vi "Vacuum Test - Step 3.vi"(7 "Step":i32, 8 "error in":errorcluster, 9 "Test Results In":T9, 10 "PAS In":T8 caption="Gas", 11 "Test Configuration":T1) -> (0 "error out":errorcluster, 1 "Test Results Out":T9, 2 "PAS Out":T8 caption="Gas", 3 "Test Configuration Out":T1)   [LabVIEW 2015]
uses:
  CAN Communication/PAS/Typedefs/Session Handle.ctl
  CAN Communication/PAS/PAS.lvclass
  Controls/Test Results.ctl
  Controls/Step Result.ctl
  Controls/Test Configuration.ctl
  Controls/Vacuum Test.ctl
  Controls/Test Timing.ctl
  Controls/Vaccum Thresholds.ctl
  Controls/Helium Test.ctl
  Controls/Helium Thresholds.ctl
  Controls/Functional Test.ctl
  CAN Communication/PAS/Typedefs/Valves.ctl
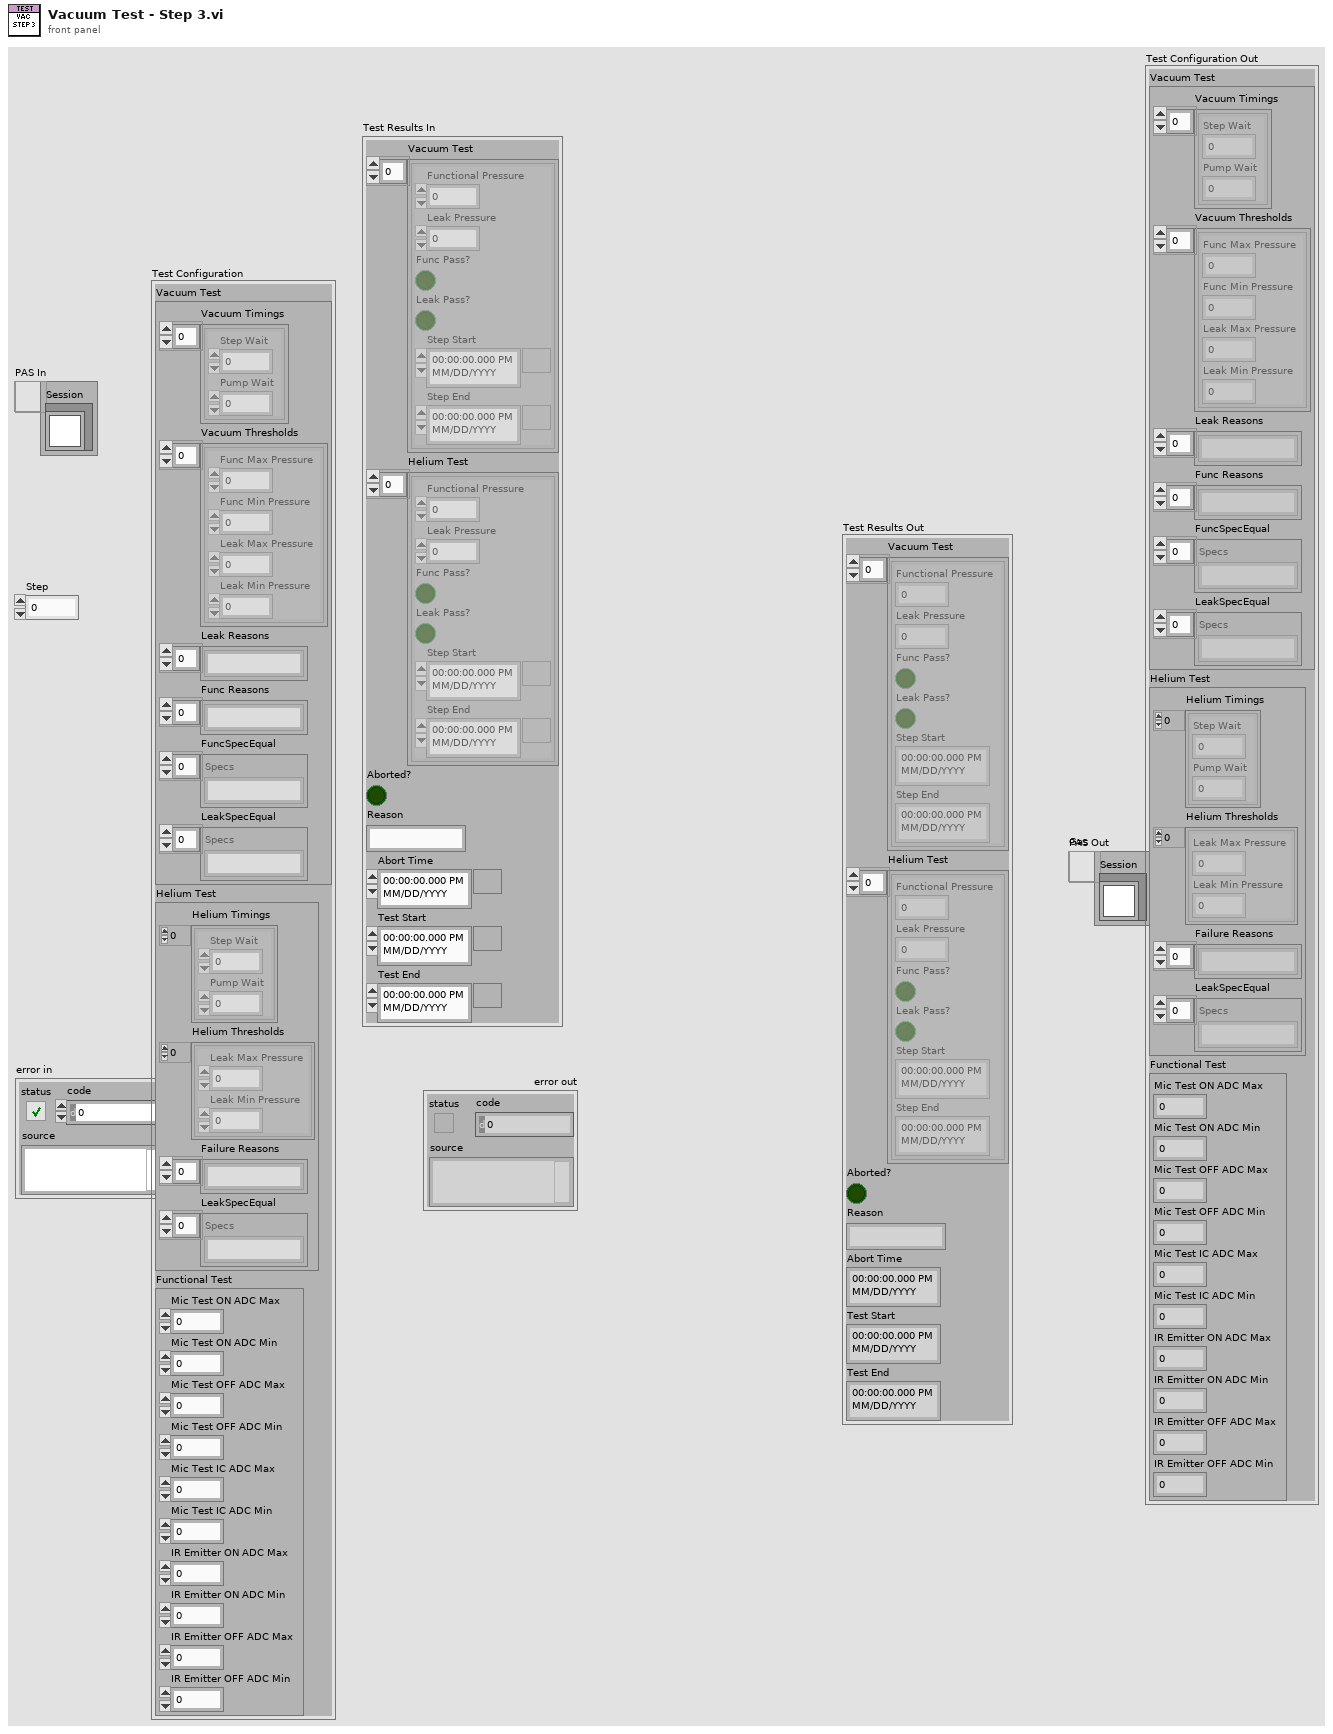
[diagram p1: front panel]
types:
  T1 = typedef "Test Configuration.ctl" = cluster{"Vacuum Test":T2, "Helium Test":T5, "Functional Test":T7}
  T2 = typedef "Vacuum Test.ctl" = cluster{"Vacuum Timings":T3[], "Vacuum Thresholds":T4[], "Leak Reasons":string[], "Func Reasons":string[], "FuncSpecEqual":string[], "LeakSpecEqual":string[]}
  T3 = typedef "Test Timing.ctl" = cluster{"Step Wait":dbl, "Pump Wait":dbl}
  T4 = typedef "Vaccum Thresholds.ctl" = cluster{"Func Max Pressure":dbl, "Func Min Pressure":dbl, "Leak Max Pressure":dbl, "Leak Min Pressure":dbl}
  T5 = typedef "Helium Test.ctl" = cluster{"Helium Timings":T3[], "Helium Thresholds":T6[], "Failure Reasons":string[], "LeakSpecEqual":string[]}
  T6 = typedef "Helium Thresholds.ctl" = cluster{"Leak Max Pressure":dbl, "Leak Min Pressure":dbl}
  T7 = typedef "Functional Test.ctl" = cluster{"Mic Test ON ADC Max":dbl, "Mic Test ON ADC Min":dbl, "Mic Test OFF ADC Max":dbl, "Mic Test OFF ADC Min":dbl, "Mic Test IC ADC Max":dbl, "Mic Test IC ADC Min":dbl, "IR Emitter ON ADC Max":dbl, "IR Emitter ON ADC Min":dbl, "IR Emitter OFF ADC Max":dbl, "IR Emitter OFF ADC Min":dbl}
  T8 = typedef "PAS.lvclass/Session Handle.ctl" = refnum<data-value>
  T9 = typedef "Test Results.ctl" = cluster{"Vacuum Test":T10[], "Helium Test":T10[], "Aborted?":bool, "Reason":string, "Abort Time":timestamp, "Test Start":timestamp, "Test End":timestamp}
  T10 = typedef "Step Result.ctl" = cluster{"Functional Pressure":dbl, "Leak Pressure":dbl, "Func Pass?":bool, "Leak Pass?":bool, "Step Start":timestamp, "Step End":timestamp}
  T11 = typedef "PAS.lvclass/Valves.ctl" = u16
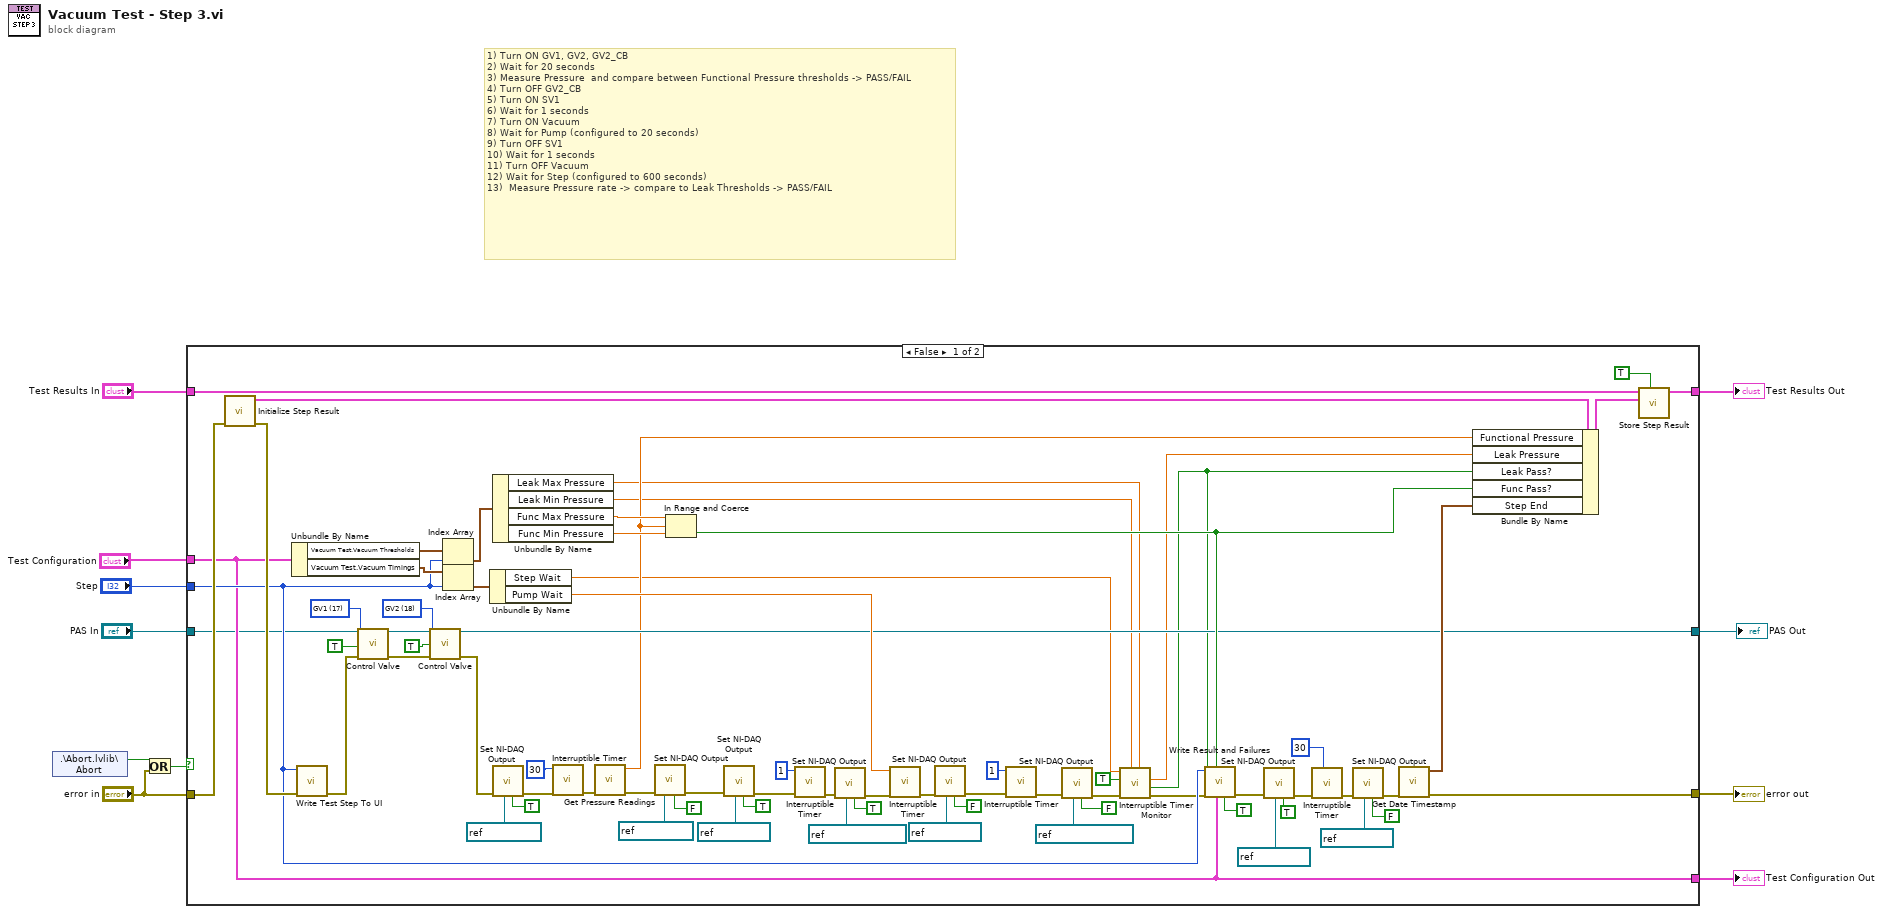
[diagram p0: block diagram]
diagram:
  # "1) Turn ON GV1, GV2, GV2_CB\n2) Wait for 20 seconds\n3) Measure Pressure  and compare between Functional Pressure thresholds -> PASS/FAIL\n4) Turn OFF GV2_CB\n5) Turn ON SV1\n6) Wait for 1 seconds\n7) Turn ON Vacuum\n8) Wait for Pump (configured to 20 seconds)\n9) Turn OFF SV1\n10) Wait for 1 seconds\n11) Turn OFF Vacuum\n12) Wait for Step (configured to 600 seconds)\n13)  Measure Pressure rate -> compare to Leak Thresholds -> PASS/FAIL"
  n1 = shared-variable ".\\Abort.lvlib\\Abort"() -> (w10:bool)  [unwired: 1 in, 1 out]
  n2 = Or(x=w10, y="error in") -> (x .or. y?=w9:bool)
  n3 = case shown="False" w9 {
    tunnel: "error in" -> [w84 w87]
    tunnel: "Test Results In" -> [w81 w88]
    tunnel: [w82 w88] -> w7
    tunnel: [w13 w87] -> w6
    tunnel: "Test Configuration" -> [w57 w86]
    tunnel: "Step" -> [w68 _]
    tunnel: [w57 w86] -> w1
    tunnel: [w32 w85] -> w3
    tunnel: "PAS In" -> [w55 w85]
    frame False {
      w47 = T11 18 items=["GV1"=17, "GV2"=18, "GV3"=19, "GV4"=20] ("Valves")
      w48 = T11 17 items=["GV1"=17, "GV2"=18, "GV3"=19, "GV4"=20] ("Valves")
      n4 = call "Initialize Step Result.vi"("error in (no error)"=w84) -> ("error out"=w83:errorcluster, "New Step Result"=w80:T10)  [unwired: 8 in, 1 out]
      n5 = Unbundle By Name(w57) -> ("Vacuum Test.Vacuum Thresholds"=w77:T4[], "Vacuum Test.Vacuum Timings"=w76:T3[])
      n6 = call "Write Test Step To UI.vi"("error in (no error)"=w83, "Step"=w68) -> ("error out"=w50:errorcluster)  [unwired: 9 in]
      n7 = call "Control Valve.vi"("Session Handle in"=w55, "Valves"=w48, "Energize?"=TRUE, "error in (no error)"=w50) -> ("Session Handle out"=w53:T8, "error out"=w51:errorcluster)  [unwired: 8 in, 2 out]
      n8 = call "Control Valve.vi"("Session Handle in"=w53, "Valves"=w47, "Energize?"=TRUE, "error in (no error)"=w51) -> ("Session Handle out"=w32:T8, "error out"=w49:errorcluster)  [unwired: 8 in, 2 out]
      n9 = Index Array(array=w77, index=w68) -> (element=w73:T4)
      n10 = Index Array(array=w76, index=w68) -> (element=w75:T3)
      n11 = Unbundle By Name(w75) -> ("Step Wait"=w29:dbl, "Pump Wait"=w41:dbl)
      n12 = Unbundle By Name(w73) -> ("Leak Max Pressure"=w27:dbl, "Leak Min Pressure"=w28:dbl, "Func Max Pressure"=w72:dbl, "Func Min Pressure"=w71:dbl)
      n13 = call "Set NI-DAQ Output.vi"("State"=TRUE, "Channel"=refnum<k21> "GV2_PAS", "error in (no error)"=w49) -> ("error out"=w66:errorcluster)  [unwired: 8 in]
      n14 = call "Interruptible Timer.vi"("error in (no error)"=w66, "Wait (s)"=30) -> ("error out"=w56:errorcluster)  [unwired: 7 in, 2 out]
      n15 = call "Get Pressure Readings.vi"("error in (no error)"=w56) -> ("error out"=w46:errorcluster, "NI-DAQ Pressure"=w31:dbl)  [unwired: 7 in, 2 out]
      n16 = call "Set NI-DAQ Output.vi"("State"=FALSE, "Channel"=refnum<k21> "GV2_PAS", "error in (no error)"=w46) -> ("error out"=w43:errorcluster)  [unwired: 8 in]
      n17 = In Range and Coerce(upper limit=w72, x=w31, lower limit=w71) -> (In Range?=w69:bool)  [unwired: 1 out]
      n18 = call "Set NI-DAQ Output.vi"("State"=TRUE, "Channel"=refnum<k21> "SV1_PAS", "error in (no error)"=w43) -> ("error out"=w61:errorcluster)  [unwired: 8 in]
      n19 = call "Interruptible Timer.vi"("error in (no error)"=w61, "Wait (s)"=1) -> ("error out"=w58:errorcluster)  [unwired: 7 in, 2 out]
      n20 = call "Set NI-DAQ Output.vi"("State"=TRUE, "Channel"=refnum<k21> "Vacuum_PAS", "error in (no error)"=w58) -> ("error out"=w42:errorcluster)  [unwired: 8 in]
      n21 = call "Interruptible Timer.vi"("error in (no error)"=w42, "Wait (s)"=w41) -> ("error out"=w34:errorcluster)  [unwired: 7 in, 2 out]
      n22 = call "Set NI-DAQ Output.vi"("State"=FALSE, "Channel"=refnum<k21> "SV1_PAS", "error in (no error)"=w34) -> ("error out"=w38:errorcluster)  [unwired: 8 in]
      n23 = call "Interruptible Timer.vi"("error in (no error)"=w38, "Wait (s)"=1) -> ("error out"=w40:errorcluster)  [unwired: 7 in, 2 out]
      n24 = call "Set NI-DAQ Output.vi"("State"=FALSE, "Channel"=refnum<k21> "Vacuum_PAS", "error in (no error)"=w40) -> ("error out"=w30:errorcluster)  [unwired: 8 in]
      n25 = call "Interruptible Timer Monitor.vi"("Max"=w27, "Min"=w28, "error in (no error)"=w30, "Update UI?"=TRUE, "Wait (s)"=w29) -> ("error out"=w15:errorcluster, "In Range?"=w25:bool, "Leak Rate"=w26:dbl)  [unwired: 3 in, 1 out]
      n26 = call "Write Result and Failures.vi"("Vacuum?"=TRUE, "Leak"=w25, "Test Configuration"=w57, "Func"=w69, "error in (no error)"=w15, "Step"=w68) -> ("error out"=w14:errorcluster)  [unwired: 5 in]
      n27 = call "Set NI-DAQ Output.vi"("State"=TRUE, "Channel"=refnum<k21> "SV1_PAS", "error in (no error)"=w14) -> ("error out"=w22:errorcluster)  [unwired: 8 in]
      n28 = call "Interruptible Timer.vi"("error in (no error)"=w22, "Wait (s)"=30) -> ("error out"=w20:errorcluster)  [unwired: 7 in, 2 out]
      n29 = call "Set NI-DAQ Output.vi"("State"=FALSE, "Channel"=refnum<k21> "SV1_PAS", "error in (no error)"=w20) -> ("error out"=w17:errorcluster)  [unwired: 8 in]
      n30 = call "Get Date Timestamp.vi"("error in (no error)"=w17) -> ("error out"=w13:errorcluster, "current time"=w78:timestamp)  [unwired: 9 in]
      n31 = Bundle By Name(cluster=w80, "Functional Pressure"=w31, "Leak Pressure"=w26, "Leak Pass?"=w25, "Func Pass?"=w69, "Step End"=w78) -> (w79:T10)
      n32 = call "Store Step Result.vi"("Vacuum?"=TRUE, "Step Result"=w79, "Test Results In"=w81) -> ("Test Results Out"=w82:T9)  [unwired: 8 in]
    }
    frame True {
    }
  }
  "error out" <- w6
  "Test Results Out" <- w7
  "PAS Out" <- w3
  "Test Configuration Out" <- w1
